vi "eLabFTW Client.vi"() -> ()   [LabVIEW 2015]
doc: "Example VI that demonstrates all library features."
uses:
  Private/Upload File to Experiment (File).vi
  Private/Upload File to Database Item (File).vi
  PL eLabFTW Client.lvclass
panel:
  in  "API key":string
  in  "server url":string="https://demo.elabftw.net"
  in  "Tab Control":T1(tab)
  in  "upload file to experiment":bool
  in  "add tag to experiment":bool
  in  "add tag to experiment parameters":cluster{"experiment id":u32, "tag":string}
  in  "add database item to experiment":bool
  in  "add database item to experiment parameters":T2
  in  "get experiment statuses":bool
  in  "experiment":T3 {"steps"."finish datetime" format="%<%X\n%x>T"; "steps"."deadline datetime" format="%<%X\n%x>T"; "files"."creation datetime" format="%<%X\n%x>T"; "last change"."datetime" format="%<%X\n%x>T"; "start datetime" format="%<%x>T"; "creation datetime" format="%<%X\n%x>T"; "last comment"."datetime" format="%<%X\n%x>T"; "timestamp"."datetime" format="%<%X\n%x>T"; "lock"."datetime" format="%<%X\n%x>T"}
  out "experiments":T4(array[cluster]) {"last comment"."datetime" format="%<%X\n%x>T"; "last change"."datetime" format="%<%X\n%x>T"; "start datetime" format="%<%X\n%x>T"}
  in  "get experiment":bool
  in  "get experiment parameters":cluster{"id":u32}
  in  "get experiments":bool
  in  "get experiments parameters":T5={"limit"=15, "offset"=0, "search string"=""}
  out "experiment statuses":T6(array[cluster])
  in  "create experiment":bool
  out "create experiment result":cluster{"new experiment id":u32}
  in  "upload file to database item":bool
  in  "create database item parameters":cluster{"type id":u32}
  in  "create database item":bool
  out "database item types":T7(array[cluster])
  in  "get database item types":bool
  in  "bookable":bool
  in  "database item":T8 {"steps"."finish datetime" format="%<%X\n%x>T"; "steps"."deadline datetime" format="%<%X\n%x>T"; "files"."creation datetime" format="%<%X\n%x>T"; "last change"."datetime" format="%<%X\n%x>T"; "start datetime" format="%<%x>T"; "last comment"."datetime" format="%<%X\n%x>T"; "lock"."datetime" format="%<%X\n%x>T"}
  in  "get database item":bool
  in  "get database item parameters":cluster{"id":u32}
  in  "get database items":bool
  in  "get datamase items parameters":T5={"limit"=15, "offset"=0, "search string"=""}
  out "database items":T9(array[cluster]) {"last comment"."datetime" format="%<%X\n%x>T"; "last change"."datetime" format="%<%X\n%x>T"; "start datetime" format="%<%X\n%x>T"}
  out "create database item result":cluster{"new item id":u32}
  in  "get template":bool
  in  "get template parameters":cluster{"id":u32}
  in  "get templates":bool
  out "templates":T10(array[cluster]) {"lock"."datetime" format="%<%X\n%x>T"}
  out "template":T11 {"lock"."datetime" format="%<%X\n%x>T"}
  out "create template result":cluster{"new template id":u32}
  in  "create template":bool
  in  "get tags":bool
  out "tags":cluster{"id":u32, "name":string}[](array[cluster])
  in  "get file":bool
  in  "get file parameters":cluster{"id":u32, "output file path":path}={"id"=0, "output file path"=path ""}
  out "file data":string
  in  "delete event":bool
  in  "delete event parameters":cluster{"id":u32}
  in  "get event":bool
  in  "get event parameters":cluster{"id":u32}
  in  "create event parameters":T12 {"end" format="%<%X\n%x>T"; "start" format="%<%X\n%x>T"}
  in  "create event":bool
  out "create event result":cluster{"new event id":u32}
  out "event":T13 {"start datetime" format="%<%X\n%x>T"; "end datetime" format="%<%X\n%x>T"}
  in  "get backup":bool
  in  "backup period":cluster{"from":timestamp, "to":timestamp} {"to" format="%<%x>T"; "from" format="%<%x>T"}
  in  "stop":bool
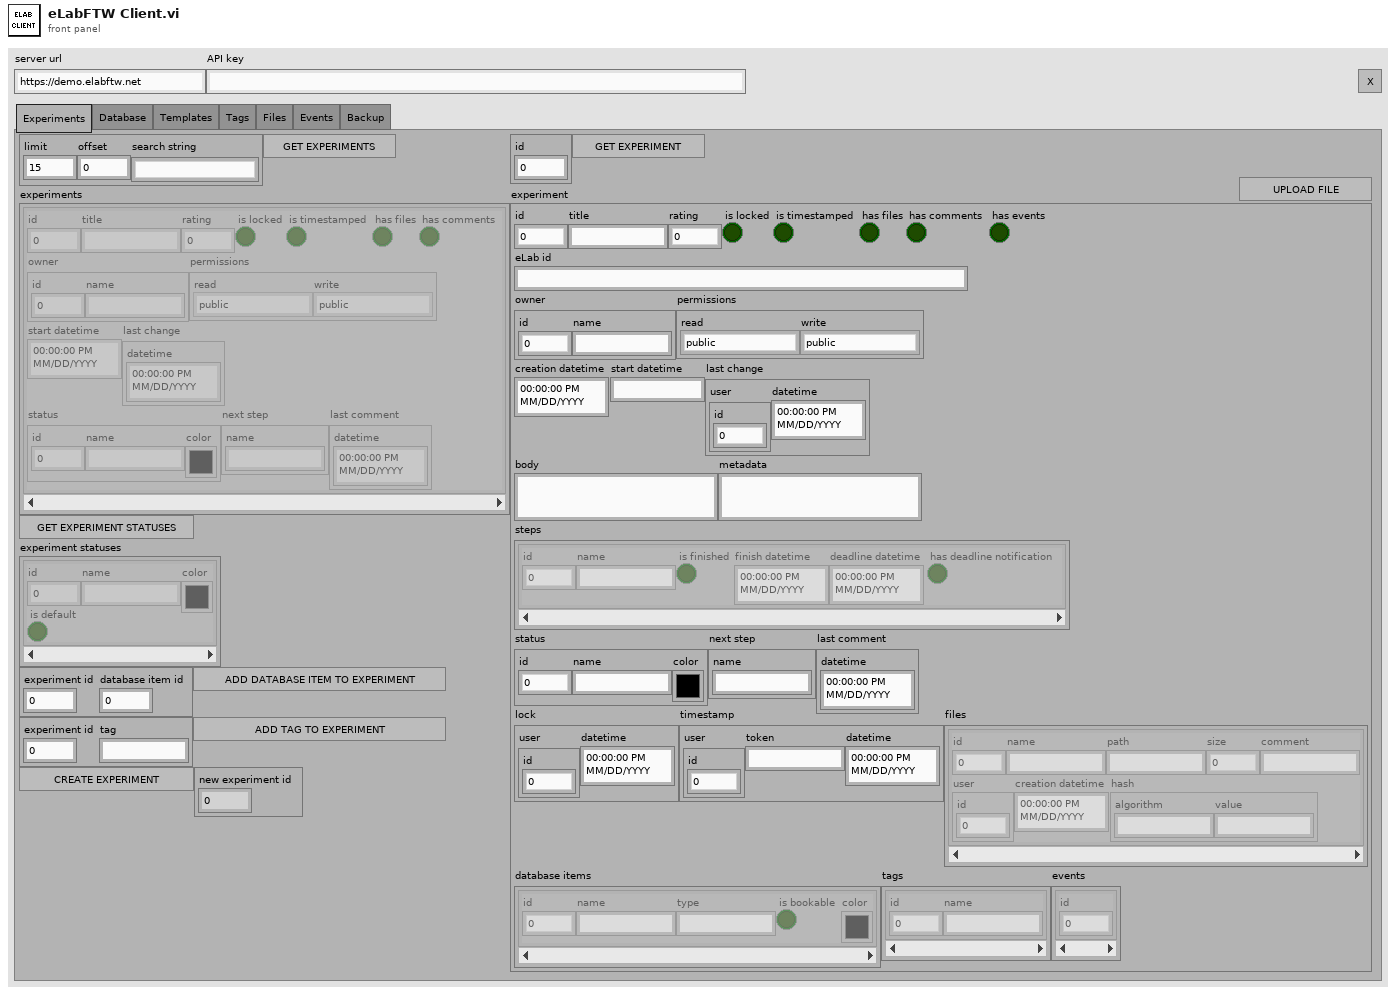
[diagram p1: front panel]
types:
  T1 = enum32{"Experiments", "Database", "Templates", "Tags", "Files", "Events", "Backup"}
  T2 = cluster{"experiment id":u32, "database item id":u32}
  T3 = cluster{"id":u32, "title":string, "rating":u32, "is locked":bool, "is timestamped":bool, "has files":bool, "has comments":bool, "has events":bool, "eLab id":string, "owner":cluster{"id":u32, "name":string}, "permissions":cluster{"read":enum16{"public", "organization", "team", "owner and admins", "owner"}, "write":enum16{"public", "organization", "team", "owner and admins", "owner"}}, "creation datetime":timestamp, "start datetime":timestamp, "last change":cluster{"user":cluster{"id":u32}, "datetime":timestamp}, "body":string, "metadata":string, "steps":cluster{"id":u32, "name":string, "is finished":bool, "finish datetime":timestamp, "deadline datetime":timestamp, "has deadline notification":bool}[], "status":cluster{"id":u32, "name":string, "color":u32}, "next step":cluster{"name":string}, "last comment":cluster{"datetime":timestamp}, "lock":cluster{"user":cluster{"id":u32}, "datetime":timestamp}, "timestamp":cluster{"user":cluster{"id":u32}, "token":string, "datetime":timestamp}, "files":cluster{"id":u32, "name":string, "path":string, "size":u32, "comment":string, "user":cluster{"id":u32}, "creation datetime":timestamp, "hash":cluster{"algorithm":string, "value":string}}[], "database items":cluster{"id":u32, "name":string, "type":string, "is bookable":bool, "color":u32}[], "tags":cluster{"id":u32, "name":string}[], "events":cluster{"id":u32}[]}
  T4 = cluster{"id":u32, "title":string, "rating":u32, "is locked":bool, "is timestamped":bool, "has files":bool, "has comments":bool, "owner":cluster{"id":u32, "name":string}, "permissions":cluster{"read":enum16{"public", "organization", "team", "owner and admins", "owner"}, "write":enum16{"public", "organization", "team", "owner and admins", "owner"}}, "start datetime":timestamp, "last change":cluster{"datetime":timestamp}, "status":cluster{"id":u32, "name":string, "color":u32}, "next step":cluster{"name":string}, "last comment":cluster{"datetime":timestamp}}[]
  T5 = cluster{"limit":u32, "offset":u32, "search string":string}
  T6 = cluster{"id":u32, "name":string, "color":u32, "is default":bool}[]
  T7 = cluster{"id":u32, "name":string, "color":u32, "is bookable":bool, "permissions":cluster{"read":enum16{"public", "organization", "team", "owner and admins", "owner"}, "write":enum16{"public", "organization", "team", "owner and admins", "owner"}}, "body":string}[]
  T8 = cluster{"id":u32, "title":string, "rating":u32, "is locked":bool, "has files":bool, "has comments":bool, "has events":bool, "is bookable":bool, "is available":bool, "eLab id":string, "owner":cluster{"id":u32, "name":string}, "team":cluster{"id":u32}, "permissions":cluster{"read":enum16{"public", "organization", "team", "owner and admins", "owner"}, "write":enum16{"public", "organization", "team", "owner and admins", "owner"}}, "start datetime":timestamp, "last change":cluster{"user":cluster{"id":u32}, "datetime":timestamp}, "body":string, "metadata":string, "steps":cluster{"id":u32, "name":string, "is finished":bool, "finish datetime":timestamp, "deadline datetime":timestamp, "has deadline notification":bool}[], "type":cluster{"id":u32, "name":string, "color":u32}, "next step":cluster{"name":string}, "last comment":cluster{"datetime":timestamp}, "lock":cluster{"user":cluster{"id":u32}, "datetime":timestamp}, "files":cluster{"id":u32, "name":string, "path":string, "size":u32, "comment":string, "user":cluster{"id":u32}, "creation datetime":timestamp, "hash":cluster{"algorithm":string, "value":string}}[], "database items":cluster{"id":u32, "name":string, "type":string, "is bookable":bool, "color":u32}[], "tags":cluster{"id":u32, "name":string}[], "events":cluster{"id":u32}[]}
  T9 = cluster{"id":u32, "title":string, "rating":u32, "is locked":bool, "has files":bool, "has comments":bool, "is bookable":bool, "owner":cluster{"id":u32, "name":string}, "permissions":cluster{"read":enum16{"public", "organization", "team", "owner and admins", "owner"}, "write":enum16{"public", "organization", "team", "owner and admins", "owner"}}, "start datetime":timestamp, "last change":cluster{"datetime":timestamp}, "type":cluster{"id":u32, "name":string, "color":u32}, "next step":cluster{"name":string}, "last comment":cluster{"datetime":timestamp}}[]
  T10 = cluster{"id":u32, "title":string, "is locked":bool, "owner":cluster{"id":u32, "name":string}, "permissions":cluster{"read":enum16{"public", "organization", "team", "owner and admins", "owner"}, "write":enum16{"public", "organization", "team", "owner and admins", "owner"}}, "body":string, "metadata":string, "lock":cluster{"user":cluster{"id":u32}, "datetime":timestamp}, "tags":cluster{"id":u32, "name":string}[]}[]
  T11 = cluster{"id":u32, "title":string, "is locked":bool, "owner":cluster{"id":u32, "name":string}, "permissions":cluster{"read":enum16{"public", "organization", "team", "owner and admins", "owner"}, "write":enum16{"public", "organization", "team", "owner and admins", "owner"}}, "body":string, "metadata":string, "lock":cluster{"user":cluster{"id":u32}, "datetime":timestamp}, "tags":cluster{"id":u32, "name":string}[]}
  T12 = cluster{"database item id":u32, "title":string, "start":timestamp, "end":timestamp}
  T13 = cluster{"id":u32, "title":string, "user":cluster{"id":u32}, "team":cluster{"id":u32}, "start datetime":timestamp, "end datetime":timestamp, "database item id":u32, "experiment id":u32}
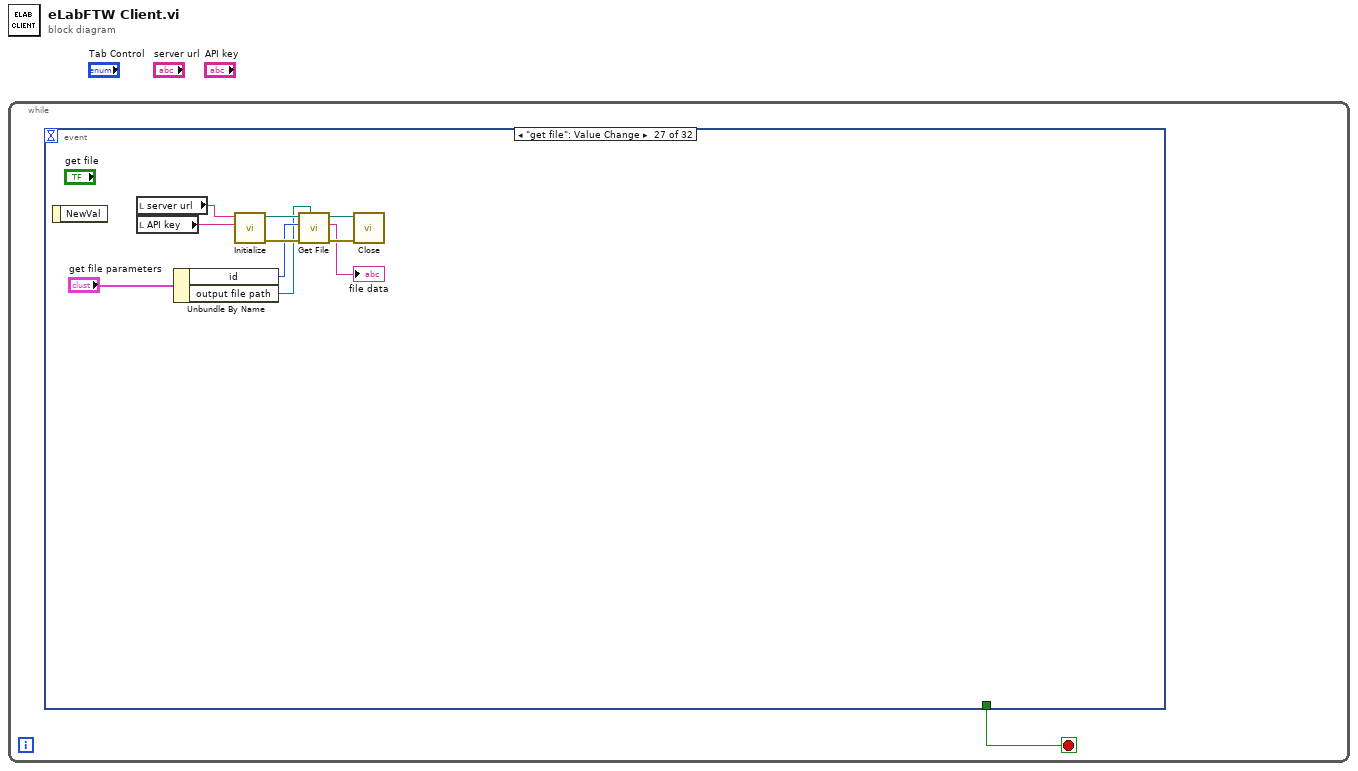
[diagram p0: block diagram]
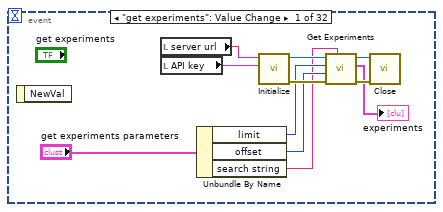
[diagram p2: hidden frame]
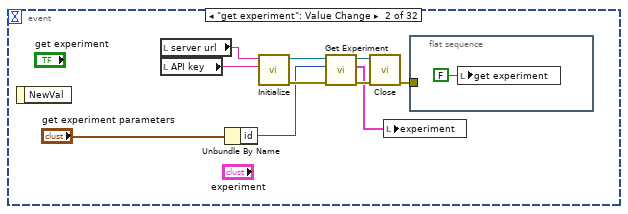
[diagram p3: hidden frame]
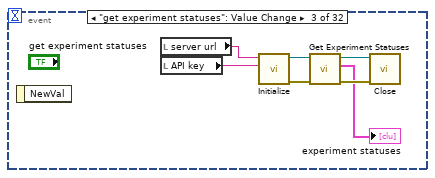
[diagram p4: hidden frame]
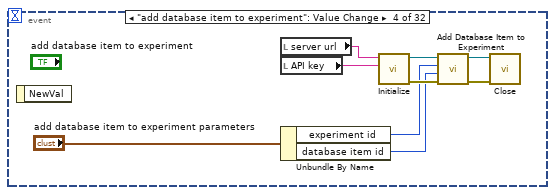
[diagram p5: hidden frame]
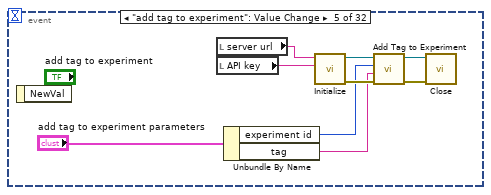
[diagram p6: hidden frame]
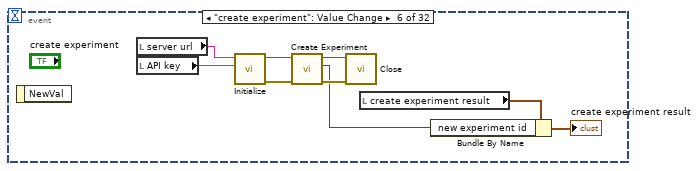
[diagram p7: hidden frame]
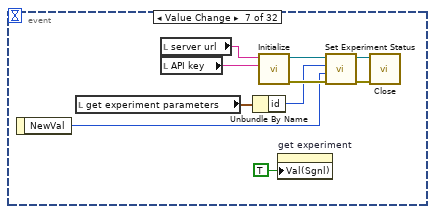
[diagram p8: hidden frame]
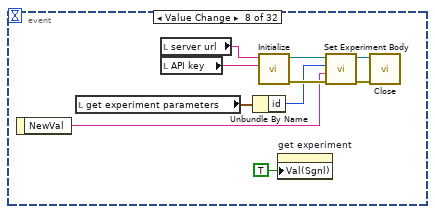
[diagram p9: hidden frame]
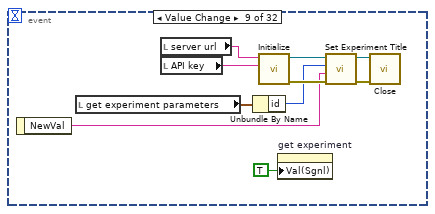
[diagram p10: hidden frame]
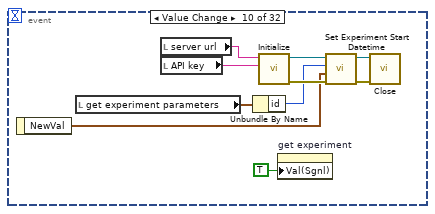
[diagram p11: hidden frame]
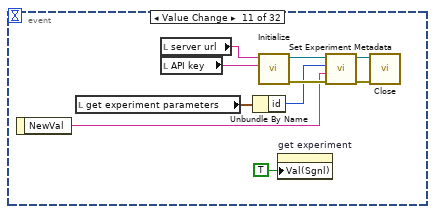
[diagram p12: hidden frame]
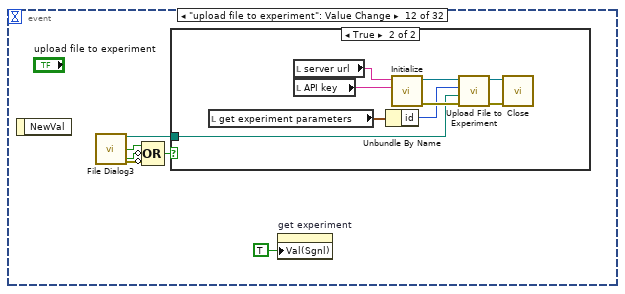
[diagram p13: hidden frame]
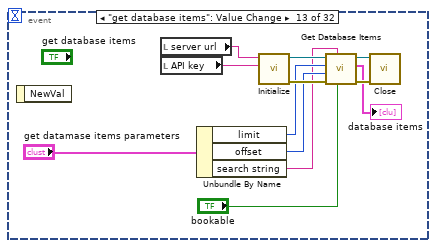
[diagram p15: hidden frame]
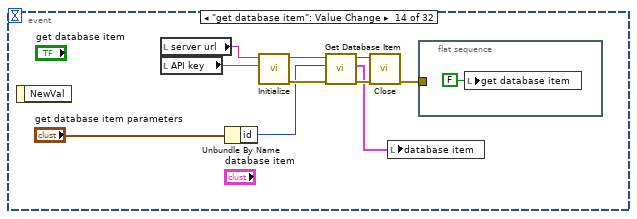
[diagram p16: hidden frame]
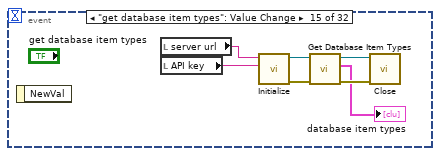
[diagram p17: hidden frame]
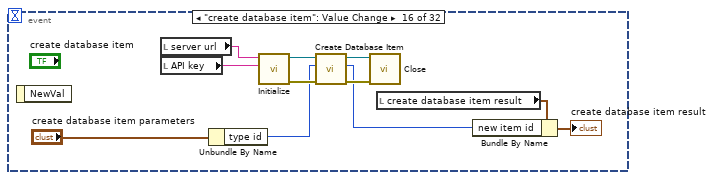
[diagram p18: hidden frame]
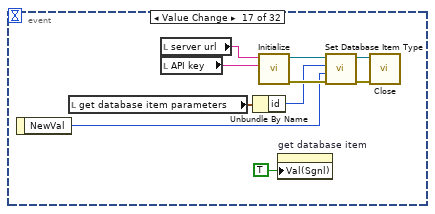
[diagram p19: hidden frame]
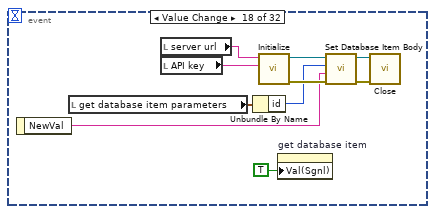
[diagram p20: hidden frame]
diagram:
  n1 = while {
    stop <- w1 stop-if-true
    n2 = event shown="[26] \"get file\": Value Change" {
      selector: _ -> [_ _ _ _ _ _ _ _ _ _ _ _ _ _ _ _ _ _ _ _ _ _ _ _ _ _ _ _ _ _ _ _]
      dyn-events: _ -> [_ _ _ _ _ _ _ _ _ _ _ _ _ _ _ _ _ _ _ _ _ _ _ _ _ _ _ _ _ _ _ _]
      timeout: _ -> [_ _ _ _ _ _ _ _ _ _ _ _ _ _ _ _ _ _ _ _ _ _ _ _ _ _ _ _ _ _ _ _]
      tunnel: [_ _ _ _ _ _ _ _ _ _ _ _ _ _ _ _ _ _ _ _ _ _ _ _ _ _ _ _ _ _ _ "stop"] -> w1
      event "get experiments": Value Change {
        n3 = event-data() -> ()  [unwired: 1 in, 1 out]
        n4 = local read "server url"() -> (w11:string)
        n5 = local read "API key"() -> (w12:string)
        n6 = Unbundle By Name("get experiments parameters") -> ("limit"=w5:u32, "offset"=w4:u32, "search string"=w3:string)
        n7 = call "Initialize.vi"("API key"=w12, "server url"=w11) -> ("error out"=w7:errorcluster, "eLab out"=w10:refnum<class "PL eLabFTW Client.lvclass">)  [unwired: 8 in]
        n8 = call "Get Experiments.vi"("search string"=w3, "error in (no error)"=w7, "offset (0)"=w4, "limit (15)"=w5, "eLab in"=w10) -> ("error out"=w8:errorcluster, "experiments"=→"experiments":T4, "eLab out"=w9:refnum<class "PL eLabFTW Client.lvclass">)  [unwired: 4 in]
        n9 = call "Close.vi"("error in (no error)"=w8, "eLab in"=w9) -> ()  [unwired: 9 in, 1 out]
      }
      event "get experiment": Value Change {
        n10 = event-data() -> ()  [unwired: 1 in, 1 out]
        n11 = local read "server url"() -> (w21:string)
        n12 = local read "API key"() -> (w22:string)
        n13 = Unbundle By Name("get experiment parameters") -> ("id"=w16:u32)
        n14 = call "Initialize.vi"("API key"=w22, "server url"=w21) -> ("error out"=w17:errorcluster, "eLab out"=w20:refnum<class "PL eLabFTW Client.lvclass">)  [unwired: 8 in]
        n15 = call "Get Experiment.vi"("error in (no error)"=w17, "id"=w16, "eLab in"=w20) -> ("error out"=w18:errorcluster, "experiment"=w14:T3, "eLab out"=w19:refnum<class "PL eLabFTW Client.lvclass">)  [unwired: 6 in]
        n16 = call "Close.vi"("error in (no error)"=w18, "eLab in"=w19) -> ("error out"=w13:errorcluster)  [unwired: 9 in]
        n17 = local write "experiment"(w14) -> ()
        n18 = flat-sequence {
          tunnel: w13 -> [_]
          frame #0 {
            n19 = local write "get experiment"(FALSE ("get experiment")) -> ()
          }
        }
      }
      event "get experiment statuses": Value Change {
        n20 = event-data() -> ()  [unwired: 1 in, 1 out]
        n21 = local read "server url"() -> (w29:string)
        n22 = local read "API key"() -> (w30:string)
        n23 = call "Initialize.vi"("API key"=w30, "server url"=w29) -> ("error out"=w25:errorcluster, "eLab out"=w28:refnum<class "PL eLabFTW Client.lvclass">)  [unwired: 8 in]
        n24 = call "Get Experiment Statuses.vi"("error in (no error)"=w25, "eLab in"=w28) -> ("error out"=w26:errorcluster, "statuses"=→"experiment statuses":T6, "eLab out"=w27:refnum<class "PL eLabFTW Client.lvclass">)  [unwired: 7 in]
        n25 = call "Close.vi"("error in (no error)"=w26, "eLab in"=w27) -> ()  [unwired: 9 in, 1 out]
      }
      event "add database item to experiment": Value Change {
        n26 = event-data() -> ()  [unwired: 1 in, 1 out]
        n27 = local read "server url"() -> (w38:string)
        n28 = local read "API key"() -> (w39:string)
        n29 = Unbundle By Name("add database item to experiment parameters") -> ("experiment id"=w32:u32, "database item id"=w31:u32)
        n30 = call "Initialize.vi"("API key"=w39, "server url"=w38) -> ("error out"=w34:errorcluster, "eLab out"=w37:refnum<class "PL eLabFTW Client.lvclass">)  [unwired: 8 in]
        n31 = call "Add Database Item to Experiment.vi"("error in (no error)"=w34, "database item id"=w31, "experiment id"=w32, "eLab in"=w37) -> ("error out"=w35:errorcluster, "eLab out"=w36:refnum<class "PL eLabFTW Client.lvclass">)  [unwired: 6 in]
        n32 = call "Close.vi"("error in (no error)"=w35, "eLab in"=w36) -> ()  [unwired: 9 in, 1 out]
      }
      event "add tag to experiment": Value Change {
        n33 = event-data() -> ()  [unwired: 1 in, 1 out]
        n34 = local read "server url"() -> (w47:string)
        n35 = local read "API key"() -> (w48:string)
        n36 = Unbundle By Name("add tag to experiment parameters") -> ("experiment id"=w42:u32, "tag"=w40:string)
        n37 = call "Initialize.vi"("API key"=w48, "server url"=w47) -> ("error out"=w43:errorcluster, "eLab out"=w46:refnum<class "PL eLabFTW Client.lvclass">)  [unwired: 8 in]
        n38 = call "Add Tag to Experiment.vi"("error in (no error)"=w43, "tag"=w40, "experiment id"=w42, "eLab in"=w46) -> ("error out"=w44:errorcluster, "eLab out"=w45:refnum<class "PL eLabFTW Client.lvclass">)  [unwired: 6 in]
        n39 = call "Close.vi"("error in (no error)"=w44, "eLab in"=w45) -> ()  [unwired: 9 in, 1 out]
      }
      event "create experiment": Value Change {
        n40 = event-data() -> ()  [unwired: 1 in, 1 out]
        n41 = local read "server url"() -> (w56:string)
        n42 = local read "API key"() -> (w57:string)
        n43 = call "Initialize.vi"("API key"=w57, "server url"=w56) -> ("error out"=w54:errorcluster, "eLab out"=w55:refnum<class "PL eLabFTW Client.lvclass">)  [unwired: 8 in]
        n44 = call "Create Experiment.vi"("error in (no error)"=w54, "eLab in"=w55) -> ("error out"=w53:errorcluster, "experiment id"=w50:u32, "eLab out"=w52:refnum<class "PL eLabFTW Client.lvclass">)  [unwired: 7 in]
        n45 = call "Close.vi"("error in (no error)"=w53, "eLab in"=w52) -> ()  [unwired: 9 in, 1 out]
        n46 = local read "create experiment result"() -> (w51:cluster{"new experiment id":u32})
        n47 = Bundle By Name(cluster=w51, "new experiment id"=w50) -> (→"create experiment result":cluster{"new experiment id":u32})
      }
      event "experiment.status.id": Value Change {
        n48 = event-data() -> ("NewVal"=w59:u32)  [unwired: 1 in]
        n49 = local read "get experiment parameters"() -> (w61:cluster{"id":u32})
        n50 = local read "server url"() -> (w66:string)
        n51 = local read "API key"() -> (w67:string)
        n52 = Unbundle By Name(w61) -> ("id"=w60:u32)
        n53 = call "Initialize.vi"("API key"=w67, "server url"=w66) -> ("error out"=w62:errorcluster, "eLab out"=w65:refnum<class "PL eLabFTW Client.lvclass">)  [unwired: 8 in]
        n54 = property on="get experiment" class="Bool (strict)"("Val(Sgnl)"=TRUE ("Value (Signaling)")) -> ()  [unwired: 2 in, 2 out]
        n55 = call "Set Experiment Status.vi"("error in (no error)"=w62, "status id"=w59, "experiment id"=w60, "eLab in"=w65) -> ("error out"=w63:errorcluster, "eLab out"=w64:refnum<class "PL eLabFTW Client.lvclass">)  [unwired: 6 in]
        n56 = call "Close.vi"("error in (no error)"=w63, "eLab in"=w64) -> ()  [unwired: 9 in, 1 out]
      }
      event "experiment.body": Value Change {
        n57 = event-data() -> ("NewVal"=w68:string)  [unwired: 1 in]
        n58 = local read "get experiment parameters"() -> (w71:cluster{"id":u32})
        n59 = local read "server url"() -> (w76:string)
        n60 = local read "API key"() -> (w77:string)
        n61 = Unbundle By Name(w71) -> ("id"=w70:u32)
        n62 = call "Initialize.vi"("API key"=w77, "server url"=w76) -> ("error out"=w72:errorcluster, "eLab out"=w75:refnum<class "PL eLabFTW Client.lvclass">)  [unwired: 8 in]
        n63 = property on="get experiment" class="Bool (strict)"("Val(Sgnl)"=TRUE ("Value (Signaling)")) -> ()  [unwired: 2 in, 2 out]
        n64 = call "Set Experiment Body.vi"("error in (no error)"=w72, "body"=w68, "experiment id"=w70, "eLab in"=w75) -> ("error out"=w73:errorcluster, "eLab out"=w74:refnum<class "PL eLabFTW Client.lvclass">)  [unwired: 6 in]
        n65 = call "Close.vi"("error in (no error)"=w73, "eLab in"=w74) -> ()  [unwired: 9 in, 1 out]
      }
      event "experiment.title": Value Change {
        n66 = event-data() -> ("NewVal"=w78:string)  [unwired: 1 in]
        n67 = local read "get experiment parameters"() -> (w81:cluster{"id":u32})
        n68 = local read "server url"() -> (w86:string)
        n69 = local read "API key"() -> (w87:string)
        n70 = Unbundle By Name(w81) -> ("id"=w80:u32)
        n71 = call "Initialize.vi"("API key"=w87, "server url"=w86) -> ("error out"=w82:errorcluster, "eLab out"=w85:refnum<class "PL eLabFTW Client.lvclass">)  [unwired: 8 in]
        n72 = property on="get experiment" class="Bool (strict)"("Val(Sgnl)"=TRUE ("Value (Signaling)")) -> ()  [unwired: 2 in, 2 out]
        n73 = call "Set Experiment Title.vi"("error in (no error)"=w82, "title"=w78, "experiment id"=w80, "eLab in"=w85) -> ("error out"=w83:errorcluster, "eLab out"=w84:refnum<class "PL eLabFTW Client.lvclass">)  [unwired: 6 in]
        n74 = call "Close.vi"("error in (no error)"=w83, "eLab in"=w84) -> ()  [unwired: 9 in, 1 out]
      }
      event "experiment.start datetime": Value Change {
        n75 = event-data() -> ("NewVal"=w88:timestamp)  [unwired: 1 in]
        n76 = local read "get experiment parameters"() -> (w91:cluster{"id":u32})
        n77 = local read "server url"() -> (w96:string)
        n78 = local read "API key"() -> (w97:string)
        n79 = Unbundle By Name(w91) -> ("id"=w90:u32)
        n80 = call "Initialize.vi"("API key"=w97, "server url"=w96) -> ("error out"=w92:errorcluster, "eLab out"=w95:refnum<class "PL eLabFTW Client.lvclass">)  [unwired: 8 in]
        n81 = property on="get experiment" class="Bool (strict)"("Val(Sgnl)"=TRUE ("Value (Signaling)")) -> ()  [unwired: 2 in, 2 out]
        n82 = call "Set Experiment Start Datetime.vi"("error in (no error)"=w92, "start datetime"=w88, "experiment id"=w90, "eLab in"=w95) -> ("error out"=w93:errorcluster, "eLab out"=w94:refnum<class "PL eLabFTW Client.lvclass">)  [unwired: 6 in]
        n83 = call "Close.vi"("error in (no error)"=w93, "eLab in"=w94) -> ()  [unwired: 9 in, 1 out]
      }
      event "experiment.metadata": Value Change {
        n84 = event-data() -> ("NewVal"=w98:string)  [unwired: 1 in]
        n85 = local read "get experiment parameters"() -> (w101:cluster{"id":u32})
        n86 = local read "server url"() -> (w106:string)
        n87 = local read "API key"() -> (w107:string)
        n88 = Unbundle By Name(w101) -> ("id"=w100:u32)
        n89 = call "Initialize.vi"("API key"=w107, "server url"=w106) -> ("error out"=w102:errorcluster, "eLab out"=w105:refnum<class "PL eLabFTW Client.lvclass">)  [unwired: 8 in]
        n90 = property on="get experiment" class="Bool (strict)"("Val(Sgnl)"=TRUE ("Value (Signaling)")) -> ()  [unwired: 2 in, 2 out]
        n91 = call "Set Experiment Metadata.vi"("error in (no error)"=w102, "metadata"=w98, "experiment id"=w100, "eLab in"=w105) -> ("error out"=w103:errorcluster, "eLab out"=w104:refnum<class "PL eLabFTW Client.lvclass">)  [unwired: 6 in]
        n92 = call "Close.vi"("error in (no error)"=w103, "eLab in"=w104) -> ()  [unwired: 9 in, 1 out]
      }
      event "upload file to experiment": Value Change {
        n93 = event-data() -> ()  [unwired: 1 in, 1 out]
        n94 = call "File Dialog3"() -> ("selected path"=w108:path, "exists"=w110:bool, "cancelled"=w111:bool, "error out"=w112:errorcluster)  [unwired: 12 in]
        n95 = Compound Arithmetic op=OR(w110, invert w111, invert w112) -> (w109:bool)
        n96 = case shown="True" w109 {
          tunnel: w108 -> [_ w114]
          frame False {
          }
          frame True {
            n97 = local read "get experiment parameters"() -> (w116:cluster{"id":u32})
            n98 = local read "server url"() -> (w121:string)
            n99 = local read "API key"() -> (w122:string)
            n100 = Unbundle By Name(w116) -> ("id"=w115:u32)
            n101 = call "Initialize.vi"("API key"=w122, "server url"=w121) -> ("error out"=w117:errorcluster, "eLab out"=w120:refnum<class "PL eLabFTW Client.lvclass">)  [unwired: 8 in]
            n102 = call-poly "Upload File to Experiment.vi"("error in (no error)"=w117, "file path"=w114, "experiment id"=w115, "eLab in"=w120) -> ("error out"=w118:errorcluster, "eLab out"=w119:refnum<class "PL eLabFTW Client.lvclass">)  [unwired: 5 in, 1 out]
            n103 = call "Close.vi"("error in (no error)"=w118, "eLab in"=w119) -> ()  [unwired: 9 in, 1 out]
          }
        }
        n104 = property on="get experiment" class="Bool (strict)"("Val(Sgnl)"=TRUE ("Value (Signaling)")) -> ()  [unwired: 2 in, 2 out]
      }
      event "get database items": Value Change {
        n105 = event-data() -> ()  [unwired: 1 in, 1 out]
        n106 = local read "server url"() -> (w133:string)
        n107 = local read "API key"() -> (w134:string)
        n108 = Unbundle By Name("get datamase items parameters") -> ("limit"=w128:u32, "offset"=w127:u32, "search string"=w126:string)
        n109 = call "Initialize.vi"("API key"=w134, "server url"=w133) -> ("error out"=w129:errorcluster, "eLab out"=w132:refnum<class "PL eLabFTW Client.lvclass">)  [unwired: 8 in]
        n110 = call "Get Database Items.vi"("bookable"="bookable", "search string"=w126, "error in (no error)"=w129, "offset (0)"=w127, "limit (15)"=w128, "eLab in"=w132) -> ("error out"=w130:errorcluster, "database items"=→"database items":T9, "eLab out"=w131:refnum<class "PL eLabFTW Client.lvclass">)  [unwired: 3 in]
        n111 = call "Close.vi"("error in (no error)"=w130, "eLab in"=w131) -> ()  [unwired: 9 in, 1 out]
      }
      event "get database item": Value Change {
        n112 = event-data() -> ()  [unwired: 1 in, 1 out]
        n113 = local read "server url"() -> (w143:string)
        n114 = local read "API key"() -> (w144:string)
        n115 = Unbundle By Name("get database item parameters") -> ("id"=w138:u32)
        n116 = call "Initialize.vi"("API key"=w144, "server url"=w143) -> ("error out"=w139:errorcluster, "eLab out"=w142:refnum<class "PL eLabFTW Client.lvclass">)  [unwired: 8 in]
        n117 = call "Get Database Item.vi"("error in (no error)"=w139, "id"=w138, "eLab in"=w142) -> ("error out"=w140:errorcluster, "database item"=w135:T8, "eLab out"=w141:refnum<class "PL eLabFTW Client.lvclass">)  [unwired: 6 in]
        n118 = call "Close.vi"("error in (no error)"=w140, "eLab in"=w141) -> ("error out"=w136:errorcluster)  [unwired: 9 in]
        n119 = local write "database item"(w135) -> ()
        n120 = flat-sequence {
          tunnel: w136 -> [_]
          frame #0 {
            n121 = local write "get database item"(FALSE ("get experiment")) -> ()
          }
        }
      }
      event "get database item types": Value Change {
        n122 = event-data() -> ()  [unwired: 1 in, 1 out]
        n123 = local read "server url"() -> (w151:string)
        n124 = local read "API key"() -> (w152:string)
        n125 = call "Initialize.vi"("API key"=w152, "server url"=w151) -> ("error out"=w147:errorcluster, "eLab out"=w150:refnum<class "PL eLabFTW Client.lvclass">)  [unwired: 8 in]
        n126 = call "Get Database Item Types.vi"("error in (no error)"=w147, "eLab in"=w150) -> ("error out"=w148:errorcluster, "types"=→"database item types":T7, "eLab out"=w149:refnum<class "PL eLabFTW Client.lvclass">)  [unwired: 7 in]
        n127 = call "Close.vi"("error in (no error)"=w148, "eLab in"=w149) -> ()  [unwired: 9 in, 1 out]
      }
      event "create database item": Value Change {
        n128 = event-data() -> ()  [unwired: 1 in, 1 out]
        n129 = local read "server url"() -> (w162:string)
        n130 = local read "API key"() -> (w163:string)
        n131 = Unbundle By Name("create database item parameters") -> ("type id"=w156:u32)
        n132 = call "Initialize.vi"("API key"=w163, "server url"=w162) -> ("error out"=w159:errorcluster, "eLab out"=w160:refnum<class "PL eLabFTW Client.lvclass">)  [unwired: 8 in]
        n133 = call "Create Database Item.vi"("error in (no error)"=w159, "type id"=w156, "eLab in"=w160) -> ("error out"=w158:errorcluster, "database item id"=w154:u32, "eLab out"=w157:refnum<class "PL eLabFTW Client.lvclass">)  [unwired: 6 in]
        n134 = call "Close.vi"("error in (no error)"=w158, "eLab in"=w157) -> ()  [unwired: 9 in, 1 out]
        n135 = local read "create database item result"() -> (w155:cluster{"new item id":u32})
        n136 = Bundle By Name(cluster=w155, "new item id"=w154) -> (→"create database item result":cluster{"new item id":u32})
      }
      event "database item.type.id": Value Change {
        n137 = event-data() -> ("NewVal"=w165:u32)  [unwired: 1 in]
        n138 = local read "get database item parameters"() -> (w167:cluster{"id":u32})
        n139 = local read "server url"() -> (w172:string)
        n140 = local read "API key"() -> (w173:string)
        n141 = Unbundle By Name(w167) -> ("id"=w166:u32)
        n142 = call "Initialize.vi"("API key"=w173, "server url"=w172) -> ("error out"=w168:errorcluster, "eLab out"=w171:refnum<class "PL eLabFTW Client.lvclass">)  [unwired: 8 in]
        n143 = property on="get database item" class="Bool (strict)"("Val(Sgnl)"=TRUE ("Value (Signaling)")) -> ()  [unwired: 2 in, 2 out]
        n144 = call "Set Database Item Type.vi"("error in (no error)"=w168, "type id"=w165, "database item id"=w166, "eLab in"=w171) -> ("error out"=w169:errorcluster, "eLab out"=w170:refnum<class "PL eLabFTW Client.lvclass">)  [unwired: 6 in]
        n145 = call "Close.vi"("error in (no error)"=w169, "eLab in"=w170) -> ()  [unwired: 9 in, 1 out]
      }
      event "database item.body": Value Change {
        n146 = event-data() -> ("NewVal"=w174:string)  [unwired: 1 in]
        n147 = local read "get database item parameters"() -> (w177:cluster{"id":u32})
        n148 = local read "server url"() -> (w182:string)
        n149 = local read "API key"() -> (w183:string)
        n150 = Unbundle By Name(w177) -> ("id"=w176:u32)
        n151 = call "Initialize.vi"("API key"=w183, "server url"=w182) -> ("error out"=w178:errorcluster, "eLab out"=w181:refnum<class "PL eLabFTW Client.lvclass">)  [unwired: 8 in]
        n152 = property on="get database item" class="Bool (strict)"("Val(Sgnl)"=TRUE ("Value (Signaling)")) -> ()  [unwired: 2 in, 2 out]
        n153 = call "Set Database Item Body.vi"("error in (no error)"=w178, "body"=w174, "database item id"=w176, "eLab in"=w181) -> ("error out"=w179:errorcluster, "eLab out"=w180:refnum<class "PL eLabFTW Client.lvclass">)  [unwired: 6 in]
        n154 = call "Close.vi"("error in (no error)"=w179, "eLab in"=w180) -> ()  [unwired: 9 in, 1 out]
      }
      event "database item.title": Value Change {
        n155 = event-data() -> ("NewVal"=w184:string)  [unwired: 1 in]
        n156 = local read "get database item parameters"() -> (w187:cluster{"id":u32})
        n157 = local read "server url"() -> (w192:string)
        n158 = local read "API key"() -> (w193:string)
        n159 = Unbundle By Name(w187) -> ("id"=w186:u32)
        n160 = call "Initialize.vi"("API key"=w193, "server url"=w192) -> ("error out"=w188:errorcluster, "eLab out"=w191:refnum<class "PL eLabFTW Client.lvclass">)  [unwired: 8 in]
        n161 = property on="get database item" class="Bool (strict)"("Val(Sgnl)"=TRUE ("Value (Signaling)")) -> ()  [unwired: 2 in, 2 out]
        n162 = call "Set Database Item Title.vi"("error in (no error)"=w188, "title"=w184, "database item id"=w186, "eLab in"=w191) -> ("error out"=w189:errorcluster, "eLab out"=w190:refnum<class "PL eLabFTW Client.lvclass">)  [unwired: 6 in]
        n163 = call "Close.vi"("error in (no error)"=w189, "eLab in"=w190) -> ()  [unwired: 9 in, 1 out]
      }
      event "database item.start datetime": Value Change {
        n164 = event-data() -> ("NewVal"=w194:timestamp)  [unwired: 1 in]
        n165 = local read "get database item parameters"() -> (w197:cluster{"id":u32})
        n166 = local read "server url"() -> (w202:string)
        n167 = local read "API key"() -> (w203:string)
        n168 = Unbundle By Name(w197) -> ("id"=w196:u32)
        n169 = call "Initialize.vi"("API key"=w203, "server url"=w202) -> ("error out"=w198:errorcluster, "eLab out"=w201:refnum<class "PL eLabFTW Client.lvclass">)  [unwired: 8 in]
        n170 = property on="get database item" class="Bool (strict)"("Val(Sgnl)"=TRUE ("Value (Signaling)")) -> ()  [unwired: 2 in, 2 out]
        n171 = call "Set Database Item Start Datetime.vi"("error in (no error)"=w198, "start datetime"=w194, "database item id"=w196, "eLab in"=w201) -> ("error out"=w199:errorcluster, "eLab out"=w200:refnum<class "PL eLabFTW Client.lvclass">)  [unwired: 6 in]
        n172 = call "Close.vi"("error in (no error)"=w199, "eLab in"=w200) -> ()  [unwired: 9 in, 1 out]
      }
      event "database item.metadata": Value Change {
        n173 = event-data() -> ("NewVal"=w204:string)  [unwired: 1 in]
        n174 = local read "get database item parameters"() -> (w207:cluster{"id":u32})
        n175 = local read "server url"() -> (w212:string)
        n176 = local read "API key"() -> (w213:string)
        n177 = Unbundle By Name(w207) -> ("id"=w206:u32)
        n178 = call "Initialize.vi"("API key"=w213, "server url"=w212) -> ("error out"=w208:errorcluster, "eLab out"=w211:refnum<class "PL eLabFTW Client.lvclass">)  [unwired: 8 in]
        n179 = property on="get database item" class="Bool (strict)"("Val(Sgnl)"=TRUE ("Value (Signaling)")) -> ()  [unwired: 2 in, 2 out]
        n180 = call "Set Database Item Metadata.vi"("error in (no error)"=w208, "metadata"=w204, "database item id"=w206, "eLab in"=w211) -> ("error out"=w209:errorcluster, "eLab out"=w210:refnum<class "PL eLabFTW Client.lvclass">)  [unwired: 6 in]
        n181 = call "Close.vi"("error in (no error)"=w209, "eLab in"=w210) -> ()  [unwired: 9 in, 1 out]
      }
      event "upload file to database item": Value Change {
        n182 = event-data() -> ()  [unwired: 1 in, 1 out]
        n183 = call "File Dialog2"() -> ("selected path"=w214:path, "exists"=w216:bool, "cancelled"=w217:bool, "error out"=w218:errorcluster)  [unwired: 12 in]
        n184 = Compound Arithmetic op=OR(w216, invert w217, invert w218) -> (w215:bool)
        n185 = case shown="True" w215 {
          tunnel: w214 -> [_ w220]
          frame False {
          }
          frame True {
            n186 = local read "get database item parameters"() -> (w222:cluster{"id":u32})
            n187 = local read "server url"() -> (w227:string)
            n188 = local read "API key"() -> (w228:string)
            n189 = Unbundle By Name(w222) -> ("id"=w221:u32)
            n190 = call "Initialize.vi"("API key"=w228, "server url"=w227) -> ("error out"=w223:errorcluster, "eLab out"=w226:refnum<class "PL eLabFTW Client.lvclass">)  [unwired: 8 in]
            n191 = call-poly "Upload File to Database Item.vi"("error in (no error)"=w223, "file path"=w220, "database item id"=w221, "eLab in"=w226) -> ("error out"=w224:errorcluster, "eLab out"=w225:refnum<class "PL eLabFTW Client.lvclass">)  [unwired: 5 in, 1 out]
            n192 = call "Close.vi"("error in (no error)"=w224, "eLab in"=w225) -> ()  [unwired: 9 in, 1 out]
          }
        }
        n193 = property on="get database item" class="Bool (strict)"("Val(Sgnl)"=TRUE ("Value (Signaling)")) -> ()  [unwired: 2 in, 2 out]
      }
      event "get templates": Value Change {
        n194 = event-data() -> ()  [unwired: 1 in, 1 out]
        n195 = local read "server url"() -> (w234:string)
        n196 = local read "API key"() -> (w235:string)
        n197 = call "Initialize.vi"("API key"=w235, "server url"=w234) -> ("error out"=w230:errorcluster, "eLab out"=w233:refnum<class "PL eLabFTW Client.lvclass">)  [unwired: 8 in]
        n198 = call "Get Templates.vi"("error in (no error)"=w230, "eLab in"=w233) -> ("error out"=w231:errorcluster, "templates"=→"templates":T10, "eLab out"=w232:refnum<class "PL eLabFTW Client.lvclass">)  [unwired: 7 in]
        n199 = call "Close.vi"("error in (no error)"=w231, "eLab in"=w232) -> ()  [unwired: 9 in, 1 out]
      }
      event "get template": Value Change {
        n200 = event-data() -> ()  [unwired: 1 in, 1 out]
        n201 = local read "server url"() -> (w243:string)
        n202 = local read "API key"() -> (w244:string)
        n203 = Unbundle By Name("get template parameters") -> ("id"=w238:u32)
        n204 = call "Initialize.vi"("API key"=w244, "server url"=w243) -> ("error out"=w239:errorcluster, "eLab out"=w242:refnum<class "PL eLabFTW Client.lvclass">)  [unwired: 8 in]
        n205 = call "Get Template.vi"("error in (no error)"=w239, "id"=w238, "eLab in"=w242) -> ("error out"=w240:errorcluster, "template"=→"template":T11, "eLab out"=w241:refnum<class "PL eLabFTW Client.lvclass">)  [unwired: 6 in]
        n206 = call "Close.vi"("error in (no error)"=w240, "eLab in"=w241) -> ()  [unwired: 9 in, 1 out]
      }
      event "create template": Value Change {
        n207 = event-data() -> ()  [unwired: 1 in, 1 out]
        n208 = local read "server url"() -> (w252:string)
        n209 = local read "API key"() -> (w253:string)
        n210 = call "Initialize.vi"("API key"=w253, "server url"=w252) -> ("error out"=w250:errorcluster, "eLab out"=w251:refnum<class "PL eLabFTW Client.lvclass">)  [unwired: 8 in]
        n211 = call "Create Template.vi"("error in (no error)"=w250, "eLab in"=w251) -> ("error out"=w249:errorcluster, "template id"=w246:u32, "eLab out"=w248:refnum<class "PL eLabFTW Client.lvclass">)  [unwired: 7 in]
        n212 = call "Close.vi"("error in (no error)"=w249, "eLab in"=w248) -> ()  [unwired: 9 in, 1 out]
        n213 = local read "create template result"() -> (w247:cluster{"new template id":u32})
        n214 = Bundle By Name(cluster=w247, "new template id"=w246) -> (→"create template result":cluster{"new template id":u32})
      }
      event "get tags": Value Change {
        n215 = event-data() -> ()  [unwired: 1 in, 1 out]
        n216 = local read "server url"() -> (w259:string)
        n217 = local read "API key"() -> (w260:string)
        n218 = call "Initialize.vi"("API key"=w260, "server url"=w259) -> ("error out"=w255:errorcluster, "eLab out"=w258:refnum<class "PL eLabFTW Client.lvclass">)  [unwired: 8 in]
        n219 = call "Get Tags.vi"("error in (no error)"=w255, "eLab in"=w258) -> ("error out"=w256:errorcluster, "tags"=→"tags":cluster{"id":u32, "name":string}[], "eLab out"=w257:refnum<class "PL eLabFTW Client.lvclass">)  [unwired: 7 in]
        n220 = call "Close.vi"("error in (no error)"=w256, "eLab in"=w257) -> ()  [unwired: 9 in, 1 out]
      }
      event "get file": Value Change {
        n221 = event-data() -> ()  [unwired: 1 in, 1 out]
        n222 = local read "server url"() -> (w265:string)
        n223 = local read "API key"() -> (w266:string)
        n224 = Unbundle By Name("get file parameters") -> ("id"=w262:u32, "output file path"=w261:path)
        n225 = call "Initialize.vi"("API key"=w266, "server url"=w265) -> ("error out"=w267:errorcluster, "eLab out"=w270:refnum<class "PL eLabFTW Client.lvclass">)  [unwired: 8 in]
        n226 = call "Get File.vi"("output file path"=w261, "error in (no error)"=w267, "id"=w262, "eLab in"=w270) -> ("error out"=w268:errorcluster, "data"=→"file data":string, "eLab out"=w269:refnum<class "PL eLabFTW Client.lvclass">)  [unwired: 5 in]
        n227 = call "Close.vi"("error in (no error)"=w268, "eLab in"=w269) -> ()  [unwired: 9 in, 1 out]
      }
      event "get event": Value Change {
        n228 = event-data() -> ()  [unwired: 1 in, 6 out]
        n229 = local read "server url"() -> (w278:string)
        n230 = local read "API key"() -> (w279:string)
        n231 = Unbundle By Name("get event parameters") -> ("id"=w273:u32)
        n232 = call "Initialize.vi"("API key"=w279, "server url"=w278) -> ("error out"=w274:errorcluster, "eLab out"=w277:refnum<class "PL eLabFTW Client.lvclass">)  [unwired: 8 in]
        n233 = call "Get Event.vi"("error in (no error)"=w274, "id"=w273, "eLab in"=w277) -> ("error out"=w275:errorcluster, "event"=→"event":T13, "eLab out"=w276:refnum<class "PL eLabFTW Client.lvclass">)  [unwired: 6 in]
        n234 = call "Close.vi"("error in (no error)"=w275, "eLab in"=w276) -> ()  [unwired: 9 in, 1 out]
      }
      event "create event": Value Change {
        n235 = event-data() -> ()  [unwired: 1 in, 1 out]
        n236 = local read "server url"() -> (w292:string)
        n237 = local read "API key"() -> (w293:string)
        n238 = Unbundle By Name("create event parameters") -> ("database item id"=w283:u32, "title"=w282:string, "start"=w281:timestamp, "end"=w280:timestamp)
        n239 = call "Initialize.vi"("API key"=w293, "server url"=w292) -> ("error out"=w290:errorcluster, "eLab out"=w291:refnum<class "PL eLabFTW Client.lvclass">)  [unwired: 8 in]
        n240 = call "Create Event.vi"("end"=w280, "start"=w281, "error in (no error)"=w290, "title"=w282, "database item id"=w283, "eLab in"=w291) -> ("error out"=w289:errorcluster, "event id"=w286:u32, "eLab out"=w288:refnum<class "PL eLabFTW Client.lvclass">)  [unwired: 3 in]
        n241 = call "Close.vi"("error in (no error)"=w289, "eLab in"=w288) -> ()  [unwired: 9 in, 1 out]
        n242 = local read "create event result"() -> (w287:cluster{"new event id":u32})
        n243 = Bundle By Name(cluster=w287, "new event id"=w286) -> (→"create event result":cluster{"new event id":u32})
      }
      event "delete event": Value Change {
        n244 = event-data() -> ()  [unwired: 1 in, 6 out]
        n245 = local read "server url"() -> (w300:string)
        n246 = local read "API key"() -> (w301:string)
        n247 = Unbundle By Name("delete event parameters") -> ("id"=w295:u32)
        n248 = call "Initialize.vi"("API key"=w301, "server url"=w300) -> ("error out"=w296:errorcluster, "eLab out"=w299:refnum<class "PL eLabFTW Client.lvclass">)  [unwired: 8 in]
        n249 = call "Delete Event.vi"("error in (no error)"=w296, "event id"=w295, "eLab in"=w299) -> ("error out"=w297:errorcluster, "eLab out"=w298:refnum<class "PL eLabFTW Client.lvclass">)  [unwired: 7 in]
        n250 = call "Close.vi"("error in (no error)"=w297, "eLab in"=w298) -> ()  [unwired: 9 in, 1 out]
      }
      event "get backup": Value Change {
        n251 = event-data() -> ()  [unwired: 1 in, 1 out]
        n252 = Unbundle By Name("backup period") -> ("from"=w312:timestamp, "to"=w311:timestamp)
        n253 = Format Into String(format string="%<%Y%m%d>T-%<%Y%m%d>T", w312, w311) -> (resulting string=w303:string)  [unwired: 2 in, 1 out]
        n254 = local read "server url"() -> (w305:string)
        n255 = local read "API key"() -> (w306:string)
        n256 = call "Initialize.vi"("API key"=w306, "server url"=w305) -> ("error out"=w307:errorcluster, "eLab out"=w310:refnum<class "PL eLabFTW Client.lvclass">)  [unwired: 8 in]
        n257 = call "Get Backup.vi"("error in (no error)"=w307, "to"=w311, "from"=w312, "eLab in"=w310) -> ("error out"=w308:errorcluster, "data"=w302:string, "eLab out"=w309:refnum<class "PL eLabFTW Client.lvclass">)  [unwired: 5 in]
        n258 = call "Close.vi"("error in (no error)"=w308, "eLab in"=w309) -> ("error out"=w304:errorcluster)  [unwired: 9 in]
        n259 = case shown="No Error" w304 {
          tunnel: w303 -> [w319 _]
          tunnel: w302 -> [w315 _]
          frame No Error {
            n260 = call "File Dialog"("default name"=w319, "pattern (all files)"="*.zip") -> ("selected path"=w316:path, "cancelled"=w318:bool, "error out"=w317:errorcluster)  [unwired: 10 in, 1 out]
            n261 = case shown="False" w318 {
              tunnel: w317 -> [w323 _]
              tunnel: w316 -> [w322 _]
              tunnel: w315 -> [w321 _]
              frame False {
                n262 = Write to Binary File(file (use dialog)=w322, data=w321, error in=w323, 5:FALSE ("prepend array or string size? (T)")) -> (refnum out=w324:refnum<file>, error out=w326:errorcluster)  [unwired: 2 in, 1 out]
                n263 = Close File(refnum=w324, error in=w326) -> ()  [unwired: 2 out]
              }
              frame True {
              }
            }
          }
          frame Error {
          }
        }
      }
      event "stop": Value Change {
        n264 = event-data() -> ()  [unwired: 1 in, 6 out]
      }
    }
  }
